vi "TEST_UI_Progress.vi"() -> ()   [LabVIEW 2021]
uses:
  Progress.lvclass
panel:
  in  "StartProgress":bool
  in  "Type":enum16{"Local Progress", "UI Progress"}(ring)
  out "error out":errorcluster
  out "Horizontal Progress Bar":u64(slide) caption="Loop 20 of 20" scale=0.0..20.0
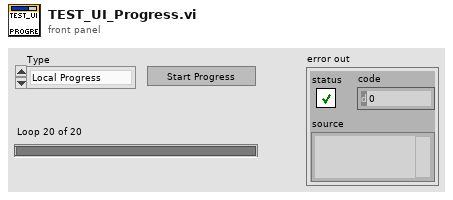
[diagram p1: front panel]
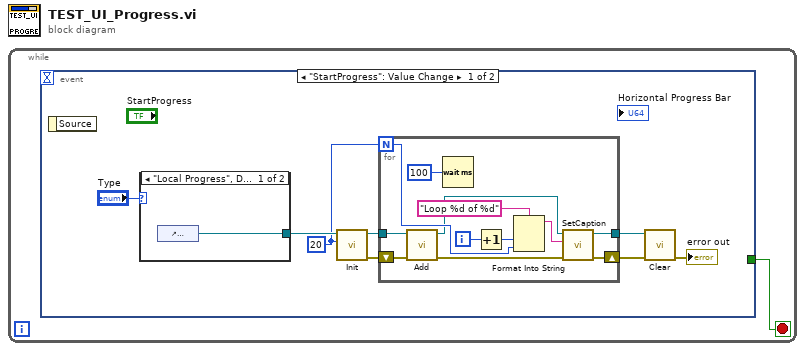
[diagram p0: block diagram]
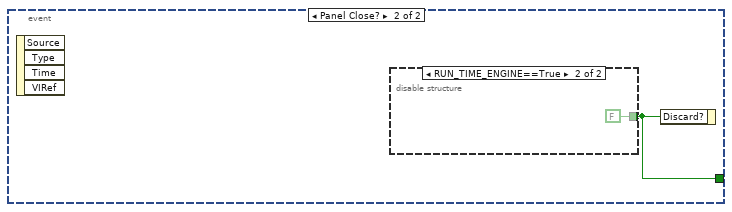
[diagram p3: hidden frame]
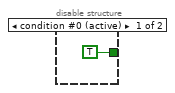
[diagram p4: hidden frame]
diagram:
  n1 = while {
    stop <- w1 stop-if-true
    n2 = event shown="[0] \"StartProgress\": Value Change" {
      selector: _ -> [_ _]
      dyn-events: _ -> [_ _]
      timeout: _ -> [_ _]
      tunnel: [_ w23] -> w1
      event "StartProgress": Value Change {
        w2 = u64 20 ("Nb Element")
        n3 = event-data() -> ()  [unwired: 1 in, 1 out]
        n4 = case shown="\"Local Progress\", Default" "Type" {
          tunnel: [w10 _] -> w3
          frame "Local Progress", Default {
            n5 = control-ref of="Horizontal Progress Bar"() -> (w10:refnum<vi>)
          }
          frame "UI Progress" {
          }
        }
        n6 = call "Init.vi"("Nb Element"=w2, "Slide Refnum"=w3) -> ("error out"=w8:errorcluster, "Progress out"=w9:refnum<class "Progress.lvclass">)  [unwired: 8 in]
        n7 = for {
          N: w2 -> [w17]
          tunnel: w9 -> [w21]
          shift-right: [w18] -> w7
          shift-left: w8 -> [w20]
          tunnel: [w11] -> w6
          i -> [w16]
          n8 = call "Add.vi"("error in (no error)"=w20, "Progress in"=w21) -> ("error out"=w19:errorcluster, "Progress out"=w12:refnum<class "Progress.lvclass">)  [unwired: 8 in]
          n9 = Wait (ms)(milliseconds to wait=u32 100) -> ()  [unwired: 1 out]
          n10 = Increment(x=w16) -> (x+1=w15:i32)
          n11 = Format Into String(format string="Loop %d of %d", w15, w17) -> (resulting string=w13:string)  [unwired: 2 in, 1 out]
          n12 = call "SetCaption.vi"("error in (no error)"=w19, "Caption"=w13, "Progress in"=w12) -> ("error out"=w18:errorcluster, "Progress out"=w11:refnum<class "Progress.lvclass">)  [unwired: 7 in]
        }
        n13 = call "Clear.vi"("error in (no error)"=w7, "Progress in"=w6) -> ("error out"=→"error out":errorcluster)  [unwired: 9 in]
      }
      event Panel Close? {
        n14 = event-data() -> ()  [unwired: 1 in, 4 out]
        n15 = disable-structure shown="RUN_TIME_ENGINE==True" {
          disable-tunnel: [TRUE FALSE] -> w23
          frame condition #0 (active) {
          }
          frame condition #1 {
          }
        }
        n16 = event-data("Discard?"=w23) -> ()  [unwired: 1 in, 1 out]
      }
    }
  }
